vi "breakIntoSampleSegements.vi"(8 "error in (no error)":errorcluster, 10 "singleToneData":T2(array[cluster]), 11 "SoundDeviceData in":refnum<class "SoundDeviceData.lvclass">) -> (0 "error out":errorcluster, 2 "segmentedData":T1(array[cluster]), 3 "SoundDeviceData out":refnum<class "SoundDeviceData.lvclass">)   [LabVIEW 2011, in "DataMappers.lvlib" / "SoundDeviceData.lvclass"]
uses:
  SoundDeviceData.lvclass
  DatabaseHelpers/Database Objects/Channel/Channel.lvclass
  SoundDeviceData.lvclass/SoundDeviceData.ctl
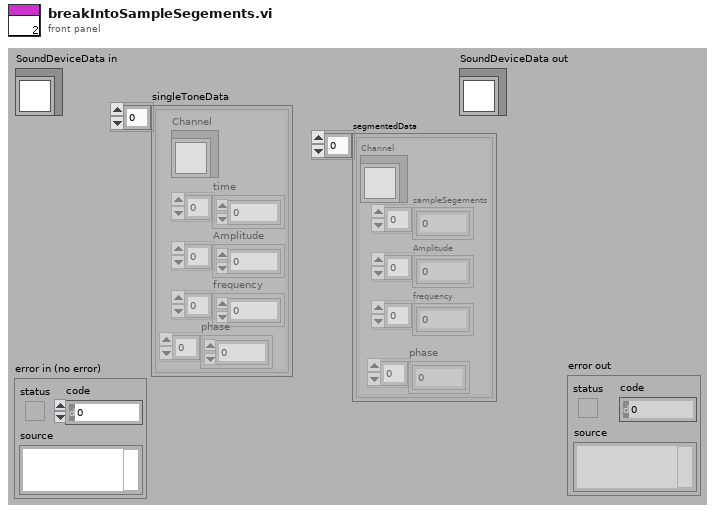
[diagram p1: front panel]
types:
  T1 = cluster{"Channel":refnum<class "Channel.lvclass">, "sampleSegements":dbl[], "Amplitude":dbl[], "frequency":dbl[], "phase":dbl[]}[]
  T2 = cluster{"Channel":refnum<class "Channel.lvclass">, "time":dbl[], "Amplitude":dbl[], "frequency":dbl[], "phase":dbl[]}[]
  T3 = cluster{"Channel":refnum<class "Channel.lvclass">, dbl[], "Amplitude":dbl[], "frequency":dbl[], "phase":dbl[]}
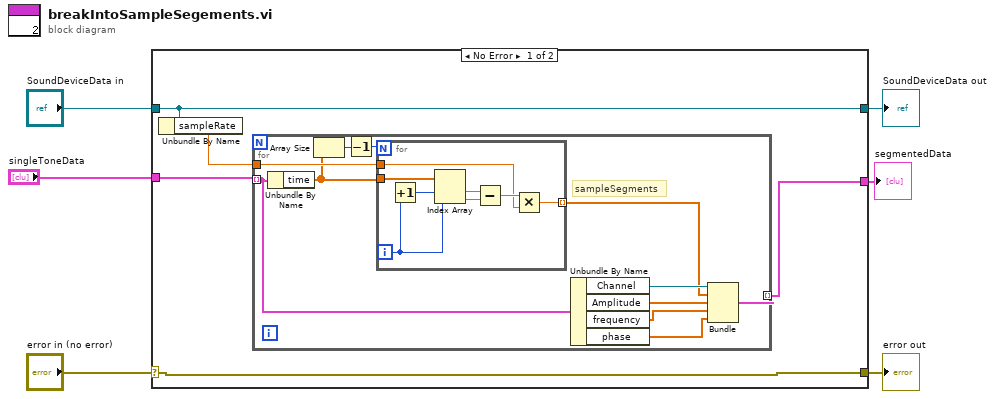
[diagram p0: block diagram]
diagram:
  n1 = case shown="No Error" "error in (no error)" {
    selector: "error in (no error)" -> [w8 w32]
    tunnel: [w8 w32] -> w5
    tunnel: [w10 w31] -> w3
    tunnel: "SoundDeviceData in" -> [w10 w31]
    tunnel: "singleToneData" -> [w11 _]
    tunnel: [w7 _] -> w1
    frame No Error {
      n2 = Unbundle By Name(w10) -> ("sampleRate"=w9:dbl)
      n3 = for {
        tunnel: w11 -> [w18] mode=indexing
        tunnel: w9 -> [w22]
        tunnel: [w13] -> w7 mode=indexing
        # "sampleSegments"
        n4 = Unbundle By Name(w18) -> ("time"=w20:dbl[])
        n5 = Array Size(array=w20) -> (size(s)=w21:i32)
        n6 = Decrement(x=w21) -> (x-1=w19:i32)
        n7 = for {
          N: w19 -> [_]
          tunnel: w22 -> [w24]
          tunnel: w20 -> [w30]
          tunnel: [w23] -> w16 mode=indexing
          i -> [w28]
          n8 = Increment(x=w28) -> (x+1=w29:i32)
          n9 = Index Array(array=w30, index #1=w29, index #2=w28) -> (element #1=w27:dbl, element #2=w26:dbl)
          n10 = Subtract(x=w27, y=w26) -> (x-y=w25:dbl)
          n11 = Multiply(x=w25, y=w24) -> (x*y=w23:dbl)
        }
        n12 = Unbundle By Name(w18) -> ("Channel"=w17:refnum<class "Channel.lvclass">, "Amplitude"=w15:dbl[], "frequency"=w14:dbl[], "phase"=w12:dbl[])
        n13 = Bundle("Channel"=w17, w16, "Amplitude"=w15, "frequency"=w14, "phase"=w12) -> (w13:T3)  [unwired: 1 in]
      }
    }
    frame Error {
    }
  }
  "error out" <- w5
  "SoundDeviceData out" <- w3
  "segmentedData" <- w1
